vi "Delete.vi"(4 "Log Map in":refnum<class "LogMap.lvclass">, 6 "commandTimeout":i32=-1, 8 "error in (no error)":errorcluster, 10 "object in":refnum<class>, 11 "SqlMapper in":refnum<class "SqlMapper.lvclass">) -> (0 "error out":errorcluster, 1 "affectedRows":i32, 3 "SqlMapper out":refnum<class "SqlMapper.lvclass">)   [LabVIEW 2020, in "ORM.lvlib" / "LogMap.lvclass"]
uses:
  LogMap.lvclass
  ORM/SqlMapper/SqlMapper.lvclass
  ORM/TypeMap/TypeMap.lvclass
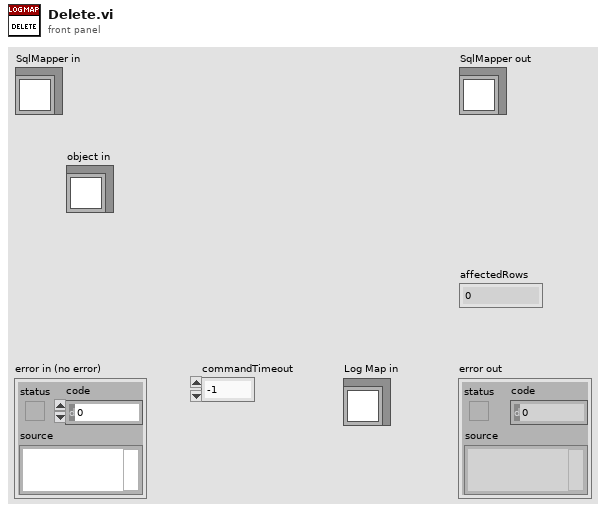
[diagram p1: front panel]
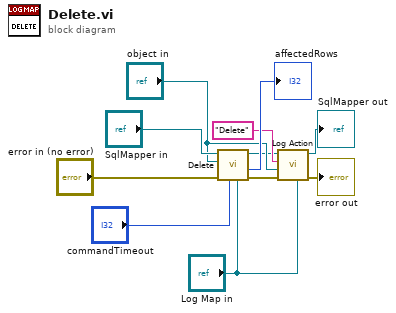
[diagram p0: block diagram]
diagram:
  n1 = call-parent "Delete.vi"("TypeMap in"="Log Map in", "commandTimeout"="commandTimeout", "error in (no error)"="error in (no error)", "object in"="object in", "SqlMapper in"="SqlMapper in") -> ("error out"=w7:errorcluster, "affectedRows"=→"affectedRows":i32, "SqlMapper out"=w2:refnum<class "SqlMapper.lvclass">)  [unwired: 4 in]
  n2 = call "Log Action.vi"("Log Map in"="Log Map in", "error in (no error)"=w7, "object in"="object in", "ActionType"="Delete", "SqlMapper in"=w2) -> ("error out"=→"error out":errorcluster, "SqlMapper out"=→"SqlMapper out":refnum<class "SqlMapper.lvclass">)  [unwired: 5 in]
